vi "Generate logfile 2.vi"(9 "Mérés":refnum<vi>, 10 "Teszt vektor listbox":refnum<vi>, 11 "Log_Path":path) -> ()   [LabVIEW 2014]
uses:
  <vilib>/Utility/file.llb/Write To Spreadsheet File (string).vi
panel:
  out "Log line":string[](array[string])
  out "Header":string[](array[string])
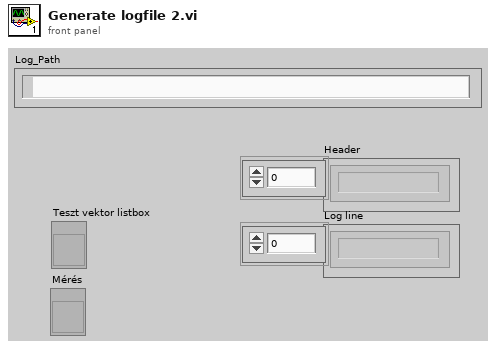
[diagram p1: front panel]
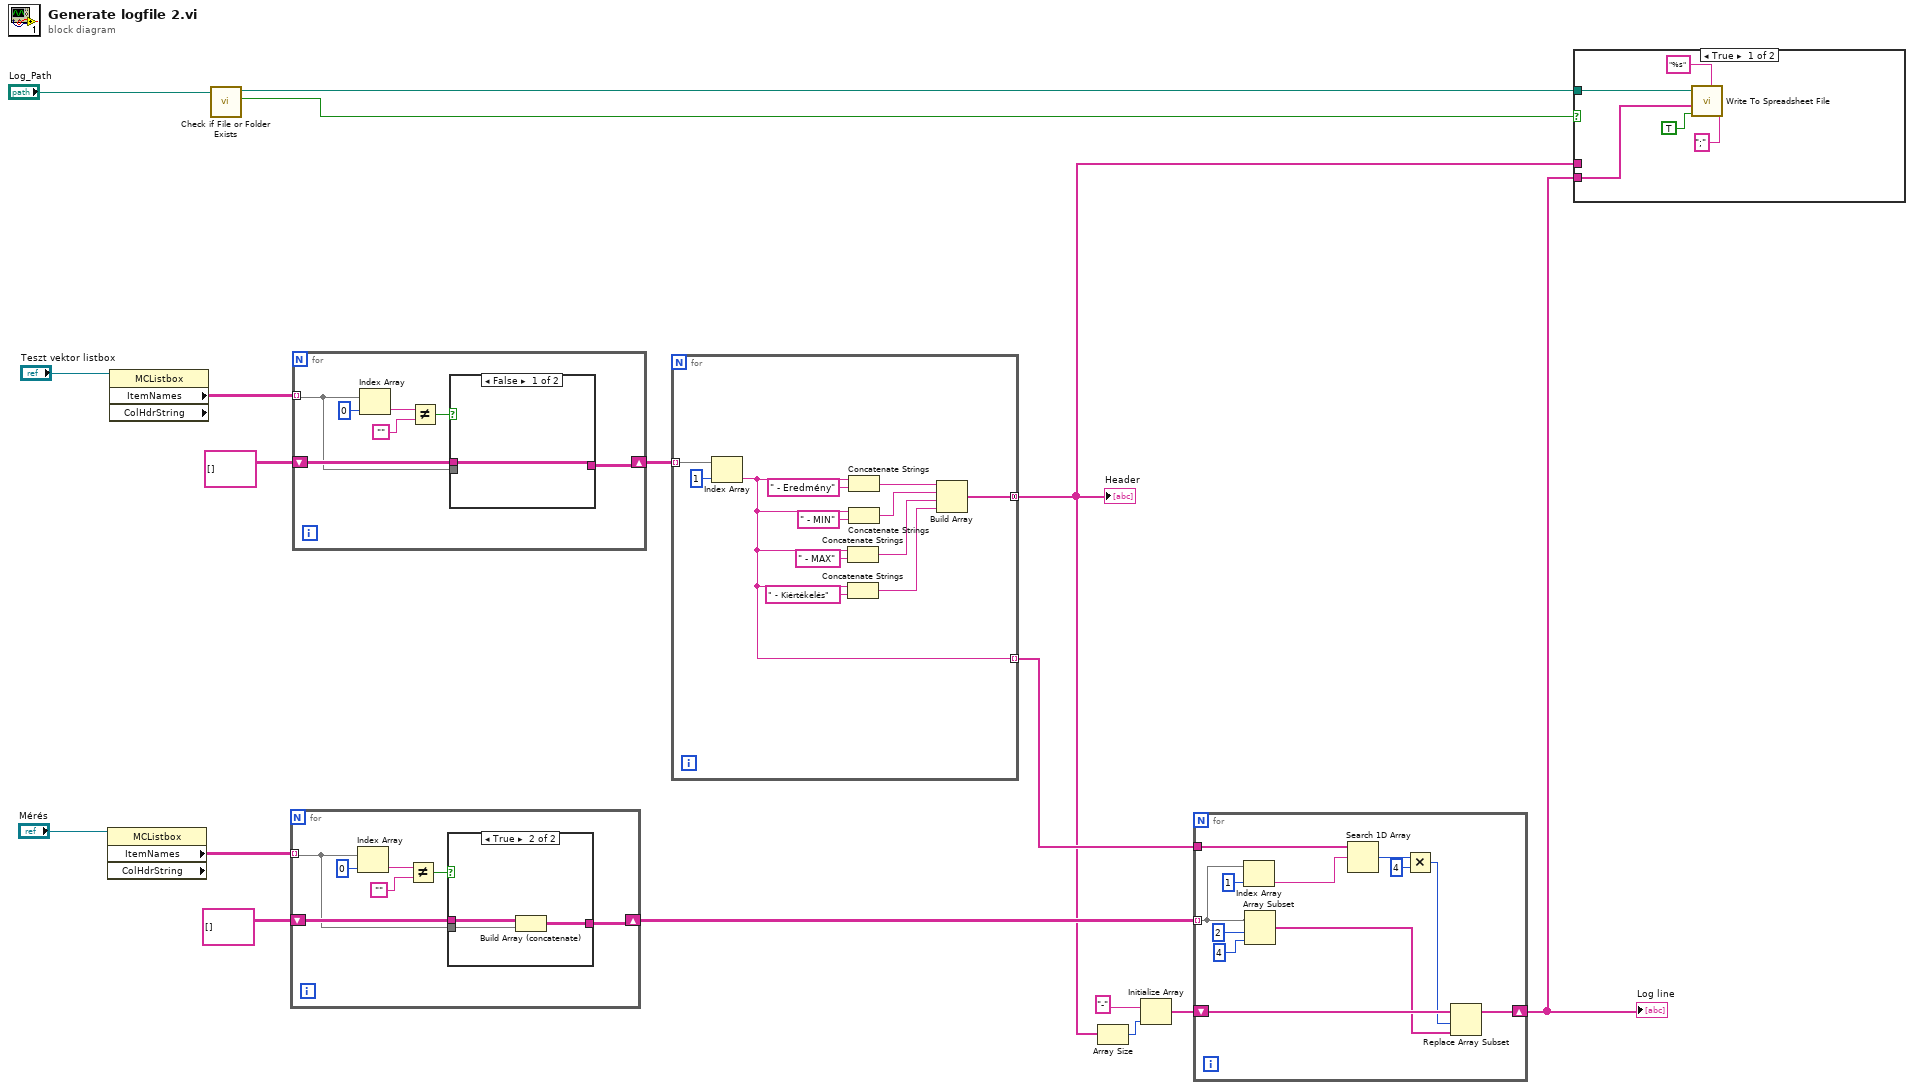
[diagram p0: block diagram]
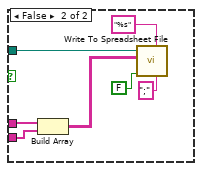
[diagram p2: hidden frame]
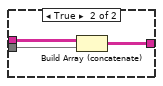
[diagram p4: hidden frame]
diagram:
  n1 = property class="MCListbox" props=["ItemNames", "ColHdrString"](reference="Mérés") -> ("ItemNames"=w12:string[][])  [unwired: 1 in, 3 out]
  n2 = property class="MCListbox" props=["ItemNames", "ColHdrString"](reference="Teszt vektor listbox") -> ("ItemNames"=w16:string[][])  [unwired: 1 in, 3 out]
  n3 = call <vilib>:"Check if File or Folder Exists.vi"("path"="Log_Path") -> ("file or folder exists?"=w9:bool, "dup path"=w8:path)  [unwired: 8 in, 1 out]
  n4 = for {
    tunnel: w12 -> [w19] mode=indexing
    shift-right: [w18] -> w7
    shift-left: string[][] [] ("Item Names") -> [w20]
    n5 = Index Array(array=w19, index=0) -> (element=w23:string)
    n6 = Not Equal?(x=w23, y="") -> (x != y?=w21:bool)
    n7 = case shown="True" w21 {
      tunnel: w20 -> [w25 w28]
      tunnel: w19 -> [_ w27]
      tunnel: [w25 w26] -> w18
      frame False {
      }
      frame True {
        n8 = Build Array (concatenate)(w28, w27) -> (w26:string[][])
      }
    }
  }
  n9 = for {
    tunnel: w16 -> [w30] mode=indexing
    shift-right: [w29] -> w14
    shift-left: string[][] [] ("Item Names") -> [w31]
    n10 = Index Array(array=w30, index=0) -> (element=w34:string)
    n11 = Not Equal?(x=w34, y="") -> (x != y?=w32:bool)
    n12 = case shown="False" w32 {
      tunnel: w31 -> [w36 w39]
      tunnel: w30 -> [_ w38]
      tunnel: [w36 w37] -> w29
      frame False {
      }
      frame True {
        n13 = Build Array (concatenate)(w39, w38) -> (w37:string[][])
      }
    }
  }
  n14 = for {
    tunnel: w14 -> [w51] mode=indexing
    tunnel: [w41] -> w3 mode=concatenating
    tunnel: [w40] -> w6 mode=indexing
    n15 = Index Array(array=w51, index=1) -> (element=w40:string)
    n16 = Concatenate Strings(w40, " - MAX" ("string")) -> (w43:string)
    n17 = Concatenate Strings(w40, " - Kiértékelés" ("string")) -> (w42:string)
    n18 = Concatenate Strings(w40, " - Eredmény" ("string")) -> (w45:string)
    n19 = Concatenate Strings(w40, " - MIN" ("string")) -> (w44:string)
    n20 = Build Array(w45, w44, w43, w42) -> (w41:string[])
  }
  "Header" <- w3
  n21 = Array Size(array=w3) -> (size(s)=w4:i32)
  n22 = Initialize Array("-", w4) -> (w2:string[])
  n23 = for {
    tunnel: w7 -> [w60] mode=indexing
    tunnel: w6 -> [w58]
    shift-right: [w52] -> w1
    shift-left: w2 -> [w55]
    n24 = Index Array(array=w60, index=1) -> (element=w59:string)
    n25 = Array Subset(array=w60, index=2, length=4) -> (w53:string[])
    n26 = Search 1D Array(1D array=w58, element=w59) -> (index of element=w57:i32)  [unwired: 1 in]
    n27 = Multiply(x=w57, y=4) -> (x*y=w54:i32)
    n28 = Replace Array Subset(array=w55, new element=w53, index=w54) -> (w52:string[])
  }
  "Log line" <- w1
  n29 = case shown="True" w9 {
    tunnel: w8 -> [w68 w75]
    tunnel: w3 -> [_ w73]
    tunnel: w1 -> [w65 w72]
    frame True {
      n30 = call-poly <vilib>:"Write To Spreadsheet File.vi"("delimiter (\\t)"=";" ("delimiter (\\t)"), "format (%s)"="%s" ("format (%.3f)"), "append to file? (new file:F)"=TRUE, "1D data"=w65, "file path (dialog if empty)"=w68) -> ()  [unwired: 3 in, 1 out]
    }
    frame False {
      n31 = Build Array(w73, w72) -> (w71:string[][])
      n32 = call-poly <vilib>:"Write To Spreadsheet File.vi"("delimiter (\\t)"=";" ("delimiter (\\t)"), "format (%s)"="%s", "append to file? (new file:F)"=FALSE, "2D data"=w71, "file path (dialog if empty)"=w75) -> ()  [unwired: 3 in, 1 out]
    }
  }
